vi "File_Parse File Name.vi"(0 "File Name":string) -> (2 "Found Extention Out":bool, 4 "File Name Out":string, 5 "Extention Out":string)   [LabVIEW 2020]
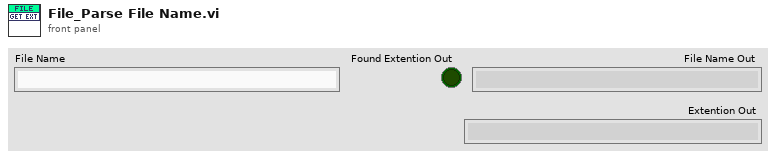
[diagram p1: front panel]
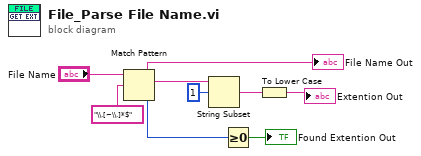
[diagram p0: block diagram]
diagram:
  n1 = Match Pattern(string="File Name", regular expression="\\.[~\\.]*$") -> (before substring=→"File Name Out":string, match substring=w3:string, offset past match=w2:i32)  [unwired: 2 out]
  n2 = String Subset(string=w3, offset (0)=1) -> (substring=w4:string)  [unwired: 1 out]
  n3 = Greater Or Equal To 0?(x=w2) -> (x >= 0?=→"Found Extention Out":bool)
  n4 = To Lower Case(string=w4) -> (all lower case string=→"Extention Out":string)
